vi "set_master_file.vi"(8 "error in (no error)":errorcluster, 11 "master file path":string) -> (0 "error out":errorcluster, 3 "master file path":path)   [LabVIEW 2017, in "worker.lvlib"]
uses:
  worker.lvlib
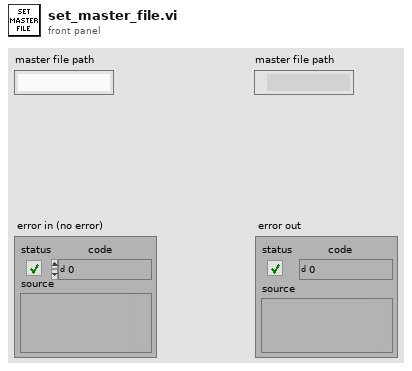
[diagram p1: front panel]
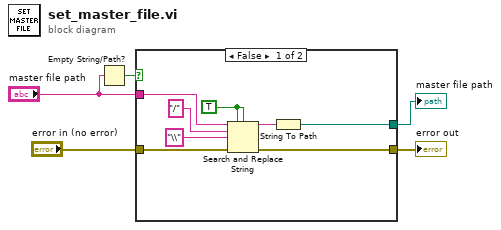
[diagram p0: block diagram]
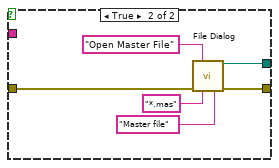
[diagram p2: hidden frame]
diagram:
  n1 = Empty String/Path?(string/path="master file path") -> (empty?=w5:bool)
  n2 = case shown="False" w5 {
    tunnel: [w13 w18] -> w3
    tunnel: "master file path" -> [w12 _]
    tunnel: "error in (no error)" -> [w7 w15]
    tunnel: [w6 w14] -> w1
    frame False {
      w9 = TRUE ("replace all? (F)")
      n3 = Search and Replace String(replace all?=w9, case sensitive?=w9, input string=w12, search string="/", replace string="\\" ("replace string (\"\")"), error in=w7) -> (result string=w8:string, error out=w6:errorcluster)  [unwired: 2 in, 2 out]
      n4 = String To Path(string=w8) -> (path=w13:path)
    }
    frame True {
      n5 = call "File Dialog"("prompt"="Open Master File", "error in"=w15, "pattern (all files)"="*.mas", "pattern label"="Master file") -> ("selected path"=w18:path, "error out"=w14:errorcluster)  [unwired: 8 in, 2 out]
    }
  }
  "error out" <- w1
  "master file path" <- w3
